vi "Add Source Node in XML.vi"(5 "Node Name":string="Source", 6 "Target":string, 7 "SourceDistribution Node":refnum<k20>, 8 "error in":errorcluster, 9 "Destination":string, 10 "Path":string, 11 "Doc Ref in":refnum<k20>) -> (0 "error out":errorcluster, 2 "Element out":refnum<k20>, 3 "Doc Ref out":refnum<k20>)   [LabVIEW 2026, in "NIVS_CDEW_MetaDataObj.lvclass"]
uses:
  NIVS_CDEW_MetaDataObj.lvclass
  NIVS_CDEW_MetaDataObj.lvclass/NIVS_CDEW_MetaDataObj.ctl
  <resource>/objmgr/DOMUserDefRef.rc
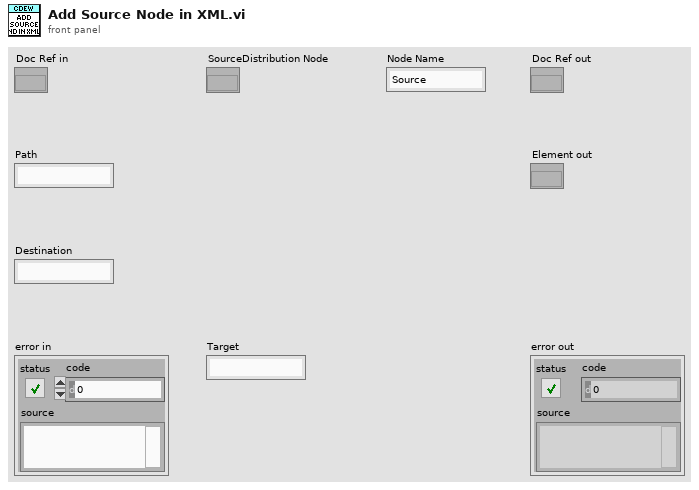
[diagram p1: front panel]
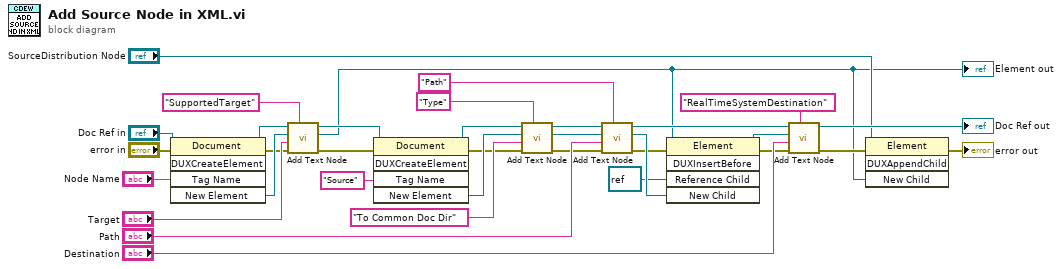
[diagram p0: block diagram]
diagram:
  n1 = invoke class="Document" method="DUXCreateElement"(reference="Doc Ref in", error in="error in", "Tag Name"="Node Name") -> (reference out=w7:refnum<k20>, error out=w6:errorcluster, "New Element"=w8:refnum<k20>)  [unwired: 2 in, 2 out]
  n2 = call "Add Text Node.vi"("Tag Name"="SupportedTarget" ("Tag Data"), "error in"=w6, "Tag Data"="Target", "Element in"=w8, "Document in"=w7) -> ("error out"=w11:errorcluster, "Element out"=w1:refnum<k20>, "Document out"=w12:refnum<k20>)  [unwired: 4 in]
  "Element out" <- w1
  n3 = invoke class="Document" method="DUXCreateElement"(reference=w12, error in=w11, "Tag Name"="Source") -> (reference out=w15:refnum<k20>, error out=w14:errorcluster, "New Element"=w16:refnum<k20>)  [unwired: 2 in, 2 out]
  n4 = call "Add Text Node.vi"("Tag Name"="Type" ("Tag Data"), "error in"=w14, "Tag Data"="To Common Doc Dir", "Element in"=w16, "Document in"=w15) -> ("error out"=w19:errorcluster, "Element out"=w21:refnum<k20>, "Document out"=w20:refnum<k20>)  [unwired: 4 in]
  n5 = call "Add Text Node.vi"("Tag Name"="Path" ("Tag Data"), "error in"=w19, "Tag Data"="Path", "Element in"=w21, "Document in"=w20) -> ("error out"=w24:errorcluster, "Element out"=w28:refnum<k20>, "Document out"=w27:refnum<k20>)  [unwired: 4 in]
  n6 = invoke class="Element" method="DUXInsertBefore"(reference=w1, error in=w24, "Reference Child"=refnum<k20> refnum, "New Child"=w28) -> (reference out=w2:refnum<k20>, error out=w26:errorcluster)  [unwired: 1 in, 3 out]
  n7 = call "Add Text Node.vi"("Tag Name"="RealTimeSystemDestination" ("Tag Data"), "error in"=w26, "Tag Data"="Destination", "Element in"=w2, "Document in"=w27) -> ("error out"=w31:errorcluster, "Document out"=→"Doc Ref out":refnum<k20>)  [unwired: 4 in, 1 out]
  n8 = invoke class="Element" method="DUXAppendChild"(reference="SourceDistribution Node", error in=w31, "New Child"=w1) -> (error out=→"error out":errorcluster)  [unwired: 1 in, 3 out]
